vi "Air Heater Model.vi"(1 "u [V]":dbl, 3 "K [C/V]":dbl=3.5, 4 "T_delay [s]":dbl=2.0, 5 "T [s]":dbl=22.0, 7 "T_env [C]":dbl=21.5, 9 "T_init [C]":dbl=21.5) -> (15 "Tout [C]":dbl)   [LabVIEW 2017]
uses:
  <vilib>/Simulation/Implementation/Shared/SIMSCR Execution Mode.ctl
  <vilib>/Simulation/Scripting/Companion Diagram/SimConfigNode/SimParams.ctl
  <vilib>/Simulation/Scripting/Companion Diagram/SimConfigNode/_simSolvers.ctl
  <vilib>/Simulation/Param Hierarchy/Typedefs/SIMPH Param Control Actions.ctl
  <vilib>/Simulation/Implementation/Shared/SIM limit type.ctl
  <vilib>/Simulation/Implementation/Shared/NILVSim_ParamChanged.vi
  <vilib>/Simulation/Implementation/Shared/NILVSIM_BeginStep.vi
  <vilib>/Simulation/ContinuousLinear/Implementation/NILVSim Integrator new.llb/SIM Integrator distributor (scalar).vi
  <vilib>/Simulation/ContinuousLinear/Implementation/NILVSim Transport Delay.llb/SIM Transport Delay Distributor (scalar).vi
  <vilib>/Simulation/ContinuousLinear/Implementation/NILVSim Transport Delay.llb/SIM Transport Delay Collector (scalar).vi
  <vilib>/Simulation/ContinuousLinear/Implementation/NILVSim Integrator new.llb/SIM Integrator collector (scalar).vi
  <vilib>/Simulation/Implementation/Shared/NILVSim_Manager.vi
  <vilib>/Utility/error.llb/Clear Errors.vi
  <vilib>/Simulation/Implementation/Shared/NILVSim_FinalizeModel.vi
  <vilib>/Simulation/Implementation/Shared/SIM Unbundle Sim Info.vi
  <vilib>/Simulation/Implementation/Shared/SIMSH Read Queue.vi
  <vilib>/Simulation/Implementation/Shared/NILVSim_Initialize.vi
  <vilib>/Simulation/Utility/Implementation/NILVSim Get Time and IsAcceptedStep.vi
  <vilib>/Simulation/Implementation/Shared/NILVSim_GetModelError.vi
  <vilib>/Simulation/Implementation/Shared/SIM SimErrorHandler.vi
  <vilib>/Simulation/Implementation/Shared/SIM Bundle Sim Info.vi
  <vilib>/Simulation/Scripting/Companion Diagram/SimConfigNode/SimDog.xnode
  <vilib>/Simulation/Implementation/XNodeFramework/SimXNode/SimX.xnode
  <vilib>/Simulation/ContinuousLinear/Implementation/NILVSim Transport Delay.llb/SIM Transport Delay Indirect (scalar).vi
  <vilib>/Simulation/ContinuousLinear/Implementation/NILVSim Integrator new.llb/SIM Integrator (scalar).vi
  <vilib>/Simulation/Implementation/Shared/NI_SIM_Implementation.lvlib
panel:
  # "Controller"
  # "Process Output"
  # "Internal Process Parameters"
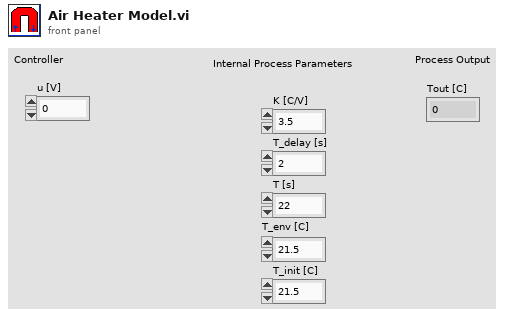
[diagram p1: front panel]
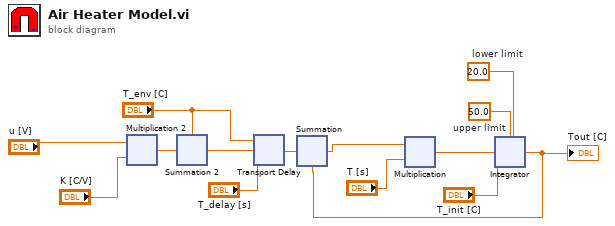
[diagram p0: block diagram]
diagram:
  w1 = 20.0  # lower limit
  w2 = 50.0  # upper limit
  n1 = xnode ("Multiplication 2")("Operand1"="u [V]", "Operand2"="K [C/V]") -> ("Result"=w6:dbl)
  n2 = xnode ("Summation 2")("Operand1"="T_env [C]", "Operand2"=w6) -> ("Result"=w5:dbl)
  n3 = xnode ("Transport Delay")("initial condition"="T_env [C]", "input"=w5, "delay (s)"="T_delay [s]") -> ("output"=w8:dbl)  [unwired: 2 in]
  n4 = xnode ("Summation")("Operand1"=w8, "Operand2"=w9) -> ("Result"=w11:dbl)
  n5 = xnode ("Multiplication")("Operand1"=w11, "Operand2"="T [s]") -> ("Result"=w13:dbl)
  n6 = xnode ("Integrator")("upper limit"=w2, "input"=w13, "initial condition"="T_init [C]", "lower limit"=w1) -> ("output"=w9:dbl)  [unwired: 6 in, 2 out]
  "Tout [C]" <- w9
